vi "get camera temperature - subvi.vi"(0 "Cooling Status In":T1) -> (1 "Cooling Status Out":T1, 2 "Error?":bool, 3 "temperature out":i32)   [LabVIEW 2014]
uses:
  lib/Andorlib/atmcd32d.lvlib
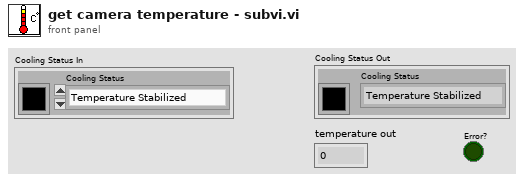
[diagram p1: front panel]
types:
  T1 = cluster{"Cooling Status":enum16{"Temperature Stabilized", "Waiting to Stabilize Temperature", "Cooling is Turned Off", "Have not yet Reached Set Temperature"}, "Color Box":u32}
  T2 = enum16{"Temperature Stabilized", "Waiting to Stabilize Temperature", "Cooling is Turned Off", "Have not yet Reached Set Temperature"}
  T3 = enum16{"Temperature Stabilized", "Waiting to Stabilize Temperature", "Cooling is Turned Off"}
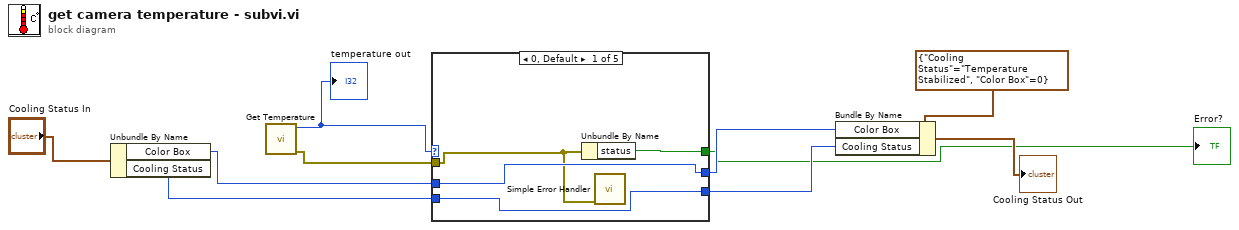
[diagram p0: block diagram]
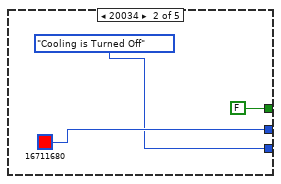
[diagram p2: hidden frame]
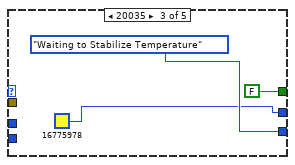
[diagram p3: hidden frame]
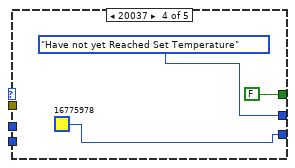
[diagram p4: hidden frame]
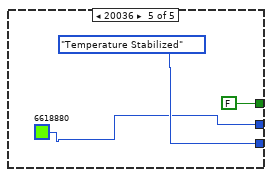
[diagram p5: hidden frame]
diagram:
  n1 = Unbundle By Name("Cooling Status In") -> ("Color Box"=w8:u32, "Cooling Status"=w7:T2)
  n2 = call "Get Temperature.vi"() -> ("error out"=w6:errorcluster, "temperature out"=w10:i32)  [unwired: 9 in, 1 out]
  "temperature out" <- w10
  n3 = case shown="0, Default" w10 {
    tunnel: [w14 FALSE ("status") FALSE ("status") FALSE ("status") FALSE ("status")] -> w1
    tunnel: [w13 u32 16711680 u32 16775978 T2."Have not yet Reached Set Temperature" ("Cooling Status") u32 6618880] -> w5
    tunnel: [w12 T3."Cooling is Turned Off" ("Cooling Status") T3."Waiting to Stabilize Temperature" ("Cooling Status") u32 16775978 T3."Temperature Stabilized" ("Cooling Status")] -> w4
    tunnel: w8 -> [w13 _ _ _ _]
    tunnel: w7 -> [w12 _ _ _ _]
    tunnel: w6 -> [w11 _ _ _ _]
    frame 0, Default {
      n4 = Unbundle By Name(w11) -> ("status"=w14:bool)
      n5 = call <vilib>:"Simple Error Handler.vi"("error in (no error)"=w11) -> ()  [unwired: 1 in, 8 out]
    }
    frame 20034 {
    }
    frame 20035 {
    }
    frame 20037 {
    }
    frame 20036 {
    }
  }
  "Error?" <- w1
  n6 = Bundle By Name(cluster=T1 {"Cooling Status"=enum."Temperature Stabilized", "Color Box"=0} ("Cooling Status 2"), "Color Box"=w5, "Cooling Status"=w4) -> (→"Cooling Status Out":T1)
